vi "Send Latching Boolean Value Change.vi"(8 "error in (no error)":errorcluster, 9 "NewVal":bool, 10 "Control Ref":refnum<vi>, 11 "Actor Enqueuer":refnum<class "Message Enqueuer.lvclass">) -> (0 "error out":errorcluster)   [LabVIEW 2015, in "LatchingBooleanValueChange.lvclass"]
uses:
  LatchingBooleanValueChange.lvclass
  <vilib>/ActorFramework/Message Enqueuer/Message Enqueuer.lvclass
  LatchingBooleanValueChange.lvclass/LatchingBooleanValueChange.ctl
  <vilib>/ActorFramework/Message Enqueuer/Message Enqueuer.lvclass/Message Enqueuer.ctl
  <vilib>/ActorFramework/Message Priority Queue/Priority Enqueue.vi
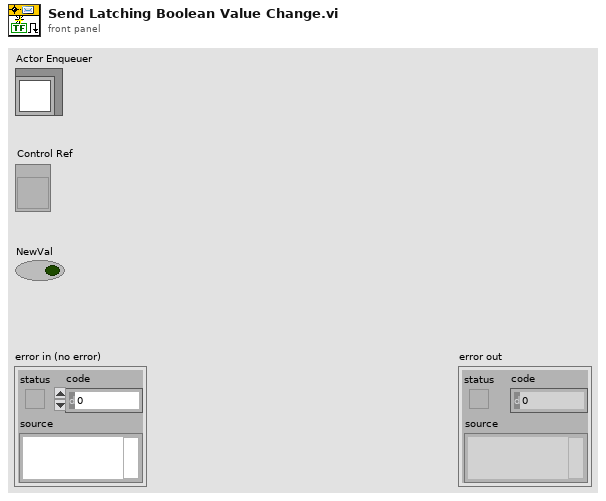
[diagram p1: front panel]
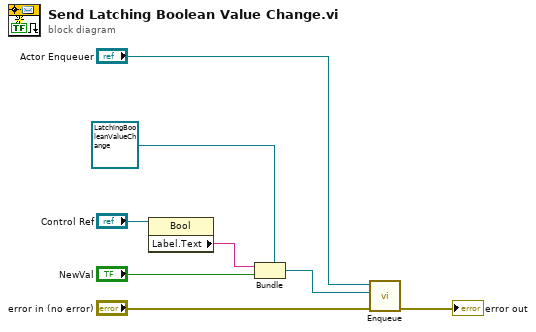
[diagram p0: block diagram]
diagram:
  n1 = property class="Bool"(reference="Control Ref") -> ("Label.Text"=w1:string)  [unwired: 1 in, 2 out]
  n2 = Bundle(cluster=refnum<class "LatchingBooleanValueChange.lvclass"> refnum ("LatchingBooleanValueChange Msg"), w1, "NewVal") -> (w6:refnum<class "LatchingBooleanValueChange.lvclass">)
  n3 = call <vilib>:"Enqueue.vi"("error in (no error)"="error in (no error)", "Message"=w6, "Message Enqueuer in"="Actor Enqueuer") -> ("error out"=→"error out":errorcluster)  [unwired: 7 in, 1 out]
